vi "Config.Gui.vi"() -> ()   [LabVIEW 2013]
uses:
  Config.Gui.Action.ctl
  CitTemplate/citTemplate.errData.ctl
  EventLog/EventLog.EventSource.ctl
  Config.Global.vi
  Global/ApplicationGlobal.vi
panel:
  in  "CancelButton":bool
  in  "SaveButton":bool
  out "_loop":i32(ring)=4
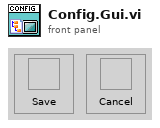
[diagram p1: front panel]
types:
  T1 = typedef "Config.Gui.Action.ctl" = enum32{"idle", "constructor", "destructor", "--- Config.Gui ---", "read from global", "write to global", "write"}
  T2 = enum32{"invalid app kind", "Development System", "Run Time System", "Student Edition", "Embedded LabVIEW", "Evaluation", "Custom"}
  T3 = typedef "citTemplate.errData.ctl" = cluster{"ts":timestamp, "src":T4, "instance":i32, "action":string, "error":errorcluster, "unconfirmed":bool}
  T4 = typedef "EventLog.EventSource.ctl" = enum16{"All", "Gui", "Ref", "File", "Seq", "Scan", "AI", "AO", "DIO", "CPX", "M1", "M2", "DB"}
  T5 = typedef "citTemplate.notifierHandle.ctl" = refnum<notifier>
  T6 = typedef "LVPositionTypeDef.ctl" = cluster{"Left":i32, "Top":i32}
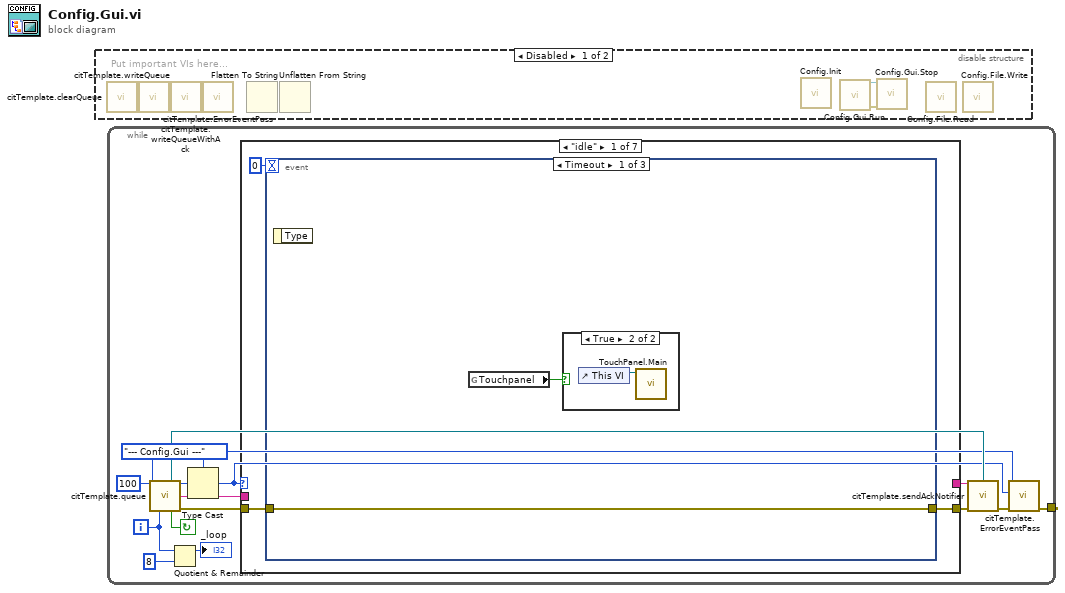
[diagram p0: block diagram]
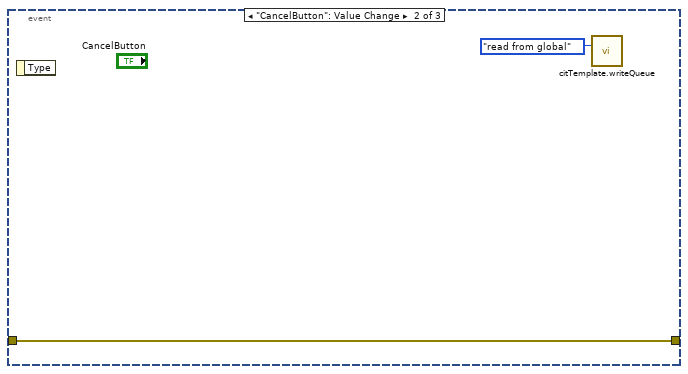
[diagram p4: hidden frame]
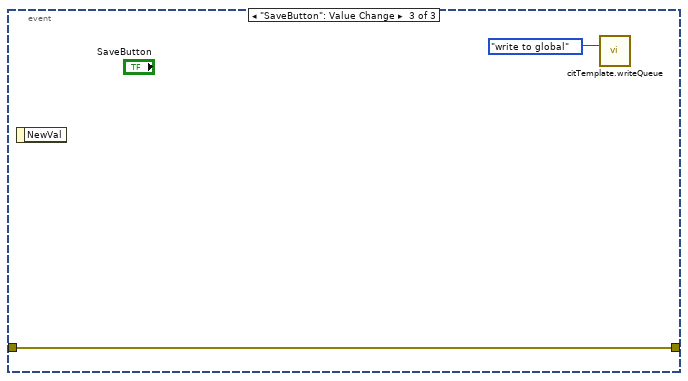
[diagram p5: hidden frame]
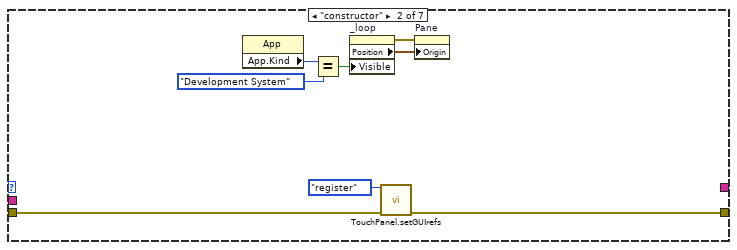
[diagram p6: hidden frame]
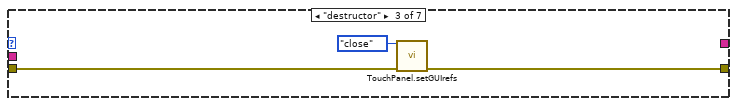
[diagram p7: hidden frame]
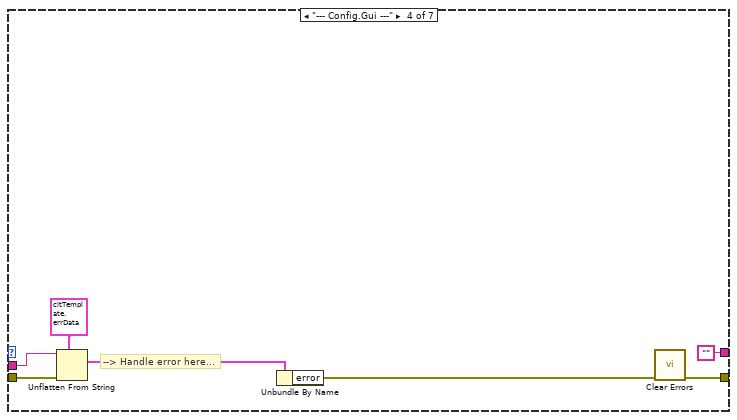
[diagram p8: hidden frame]
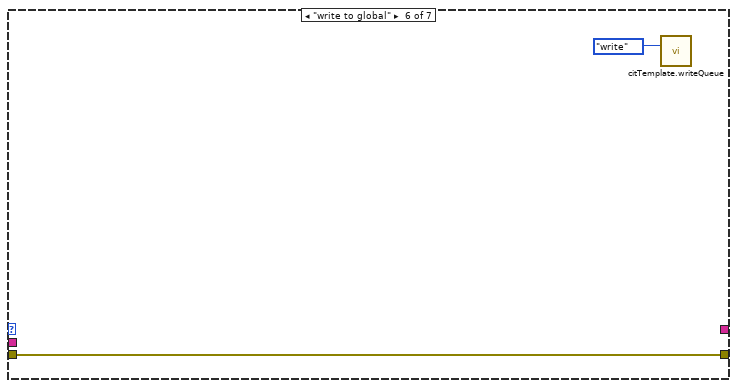
[diagram p10: hidden frame]
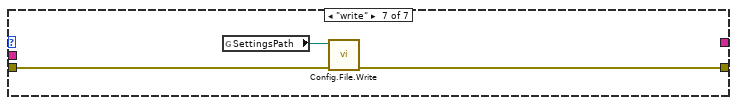
[diagram p11: hidden frame]
diagram:
  n1 = disable-structure shown="Disabled" {
    frame Disabled {
      # "Put important VIs here..."
      n2 = call "citTemplate.clearQueue.vi"() -> ()  [unwired: 14 in, 2 out]
      n3 = call "citTemplate.writeQueue.vi"() -> ()  [unwired: 15 in, 1 out]
      n4 = call "citTemplate.writeQueueWithAck.vi"() -> ()  [unwired: 13 in, 3 out]
      n5 = call "citTemplate.ErrorEventPass.vi"() -> ()  [unwired: 11 in, 1 out]
      n6 = Flatten To String() -> ()  [unwired: 4 in, 3 out]
      n7 = Unflatten From String() -> ()  [unwired: 5 in, 3 out]
      n8 = call "Config.Init.vi"() -> ()  [unwired: 11 in, 1 out]
      n9 = call "Config.Gui.Run.vi"() -> ("error out"=w2:errorcluster, "Ref"=w1:refnum<vi>)  [unwired: 10 in]
      n10 = call "Config.Gui.Stop.vi"("error in"=w2, "Ref"=w1) -> ()  [unwired: 9 in, 1 out]
      n11 = call "Config.File.Read.vi"() -> ()  [unwired: 11 in, 1 out]
      n12 = call "Config.File.Write.vi"() -> ()  [unwired: 11 in, 1 out]
    }
    frame Enabled {
    }
  }
  n13 = while {
    tunnel: [w3] -> _
    i -> [w10]
    stop <- w13 continue-if-true
    w5 = Config.Gui.Action."--- Config.Gui ---" ("Action")
    n14 = call "citTemplate.queue.vi"("ms timeout (250 ms)"=100, "event enum"=w5, "iteration (-1)"=w10) -> ("notifierHandle out"=w8:T5, "event out"=w16:u32, "(flatten) data out"=w15:string, "continue"=w13:bool, "error out"=w14:errorcluster)  [unwired: 2 in, 6 out]
    n15 = Quotient & Remainder(x=w10, y=8) -> (x-y*floor(x/y)=→"_loop":i32)  [unwired: 1 out]
    n16 = Type Cast(type=w5, x=w16) -> (*(type *) &x=w4:T1)
    n17 = case shown="\"idle\"" w4 {
      tunnel: w15 -> [_ _ _ w44 _ _ _]
      tunnel: w14 -> [w18 w33 w36 w43 w45 w46 w50]
      tunnel: [w17 w32 w35 w41 w45 w46 w48] -> w6
      tunnel: [_ _ _ "" _ _ _] -> w7
      frame "idle" {
        n18 = event shown="[0] Timeout" {
          selector: _ -> [_ _ _]
          dyn-events: _ -> [_ _ _]
          timeout: 0 -> [_ _ _]
          tunnel: [w21 w23 w25] -> w17
          tunnel: w18 -> [w21 w23 w25]
          event Timeout {
            n19 = event-data() -> ()  [unwired: 1 in, 1 out]
            n20 = global read "Config.Global.vi" "Touchpanel"() -> (w20:bool)
            n21 = case shown="True" w20 {
              frame False {
              }
              frame True {
                n22 = control-ref of="This VI"() -> (w22:refnum<vi>)
                n23 = call "TouchPanel.Main.vi"("VI ref"=w22) -> ()  [unwired: 9 in, 2 out]
              }
            }
          }
          event "CancelButton": Value Change {
            n24 = event-data() -> ()  [unwired: 1 in, 1 out]
            n25 = call "citTemplate.writeQueue.vi"("event in (if not connected:all statemachine with data event)"=Config.Gui.Action."read from global" ("Action")) -> ()  [unwired: 14 in, 1 out]
          }
          event "SaveButton": Value Change {
            n26 = event-data() -> ()  [unwired: 1 in, 1 out]
            n27 = call "citTemplate.writeQueue.vi"("event in (if not connected:all statemachine with data event)"=Config.Gui.Action."write to global" ("Action")) -> ()  [unwired: 14 in, 1 out]
          }
        }
      }
      frame "constructor" {
        n28 = property class="App"() -> ("App.Kind"=w29:T2)  [unwired: 2 in, 2 out]
        n29 = Equal?(x=w29, y=T2."Development System") -> (x = y?=w27:bool)
        n30 = property on="_loop" class="Ring (strict)"("Visible"=w27) -> (error out=w31:errorcluster, "Position"=w30:T6)  [unwired: 2 in, 1 out]
        n31 = call "TouchPanel.setGUIrefs.vi"("register mode (close & register)"=enum16{"close & register", "register", "close"}."register", "error in (no error)"=w33) -> ("dup of error in"=w32:errorcluster)  [unwired: 12 in, 1 out]
        n32 = property on="Pane" class="Pane"(error in=w31, "Origin"=w30) -> ()  [unwired: 1 in, 2 out]
      }
      frame "destructor" {
        n33 = call "TouchPanel.setGUIrefs.vi"("register mode (close & register)"=enum16{"close & register", "register", "close"}."close", "error in (no error)"=w36) -> ("dup of error in"=w35:errorcluster)  [unwired: 12 in, 1 out]
      }
      frame "--- Config.Gui ---" {
        # "--> Handle error here..."
        n34 = Unflatten From String(type=T3 {"ts"=timestamp(0 s since 1904-01-01), "src"=enum."All", "instance"=0, "action"="", "error"={"status"=FALSE, "code"=0, "source"=""}, "unconfirmed"=FALSE} ("ErrData"), binary string=w44, error in (no error)=w43) -> (value=w42:T3)  [unwired: 4 out]
        n35 = Unbundle By Name(w42) -> ("error"=w38:errorcluster)
        n36 = call <vilib>:"Clear Errors.vi"("error in (no error)"=w38) -> ("error out"=w41:errorcluster)  [unwired: 6 in]
      }
      frame "read from global" {
      }
      frame "write to global" {
        n37 = call "citTemplate.writeQueue.vi"("event in (if not connected:all statemachine with data event)"=Config.Gui.Action."write" ("Action")) -> ()  [unwired: 14 in, 1 out]
      }
      frame "write" {
        n38 = global read "ApplicationGlobal.vi" "SettingsPath"() -> (w49:path)
        n39 = call "Config.File.Write.vi"("error in"=w50, "path"=w49) -> ("error out"=w48:errorcluster)  [unwired: 9 in]
      }
    }
    n40 = call "citTemplate.sendAckNotifier.vi"("notification data"=w7, "notifierHandle in"=w8, "error in"=w6) -> ()  [unwired: 13 in]
    n41 = call "citTemplate.ErrorEventPass.vi"("error in"=w6, "action of error"=w4, "event in"=w5) -> ("error out"=w3:errorcluster)  [unwired: 8 in]
  }
